vi "Data.vi"(11 "Error Msg Strategy in":refnum<class "Error Msg Strategy.lvclass">) -> (2 "Error":errorcluster)   [LabVIEW 2021, in "Error.lvlib" / "Error Msg Strategy.lvclass"]
uses:
  Error Msg Strategy.lvclass
  Error Msg Strategy.lvclass/Error Msg Strategy.ctl
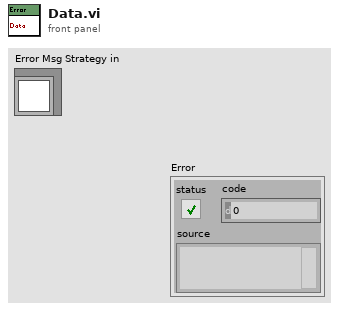
[diagram p1: front panel]
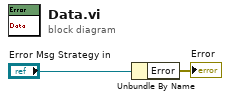
[diagram p0: block diagram]
diagram:
  n1 = Unbundle By Name("Error Msg Strategy in") -> ("Error"=→"Error":errorcluster)
